vi "Get Default Value.vi"(8 "error in":errorcluster, 9 "project refnum":refnum<vi>, 10 "measurement_signature":T2, 11 "gRPCid in":T1) -> (0 "error out":errorcluster, 3 "default value":variant)   [LabVIEW 2021, in "MeasurementClient Editor.lvlib"]
uses:
  MeasurementClient Editor.lvlib
  <vilib>/gRPC/Generated APIs/ni/measurementlink/measurement/v2/Measurement Service Client V2/RPC Messages/ni_measurementlink_measurement_v2_MeasurementSignature.ctl
  <vilib>/gRPC/Generated APIs/ni/measurementlink/measurement/v2/Measurement Service Client V2/RPC Messages/ni_measurementlink_measurement_v2_ConfigurationParameter.ctl
  <vilib>/gRPC/Generated APIs/ni/measurementlink/measurement/v2/Measurement Service Client V2/RPC Messages/google_protobuf_Field_Kind.ctl
  <vilib>/gRPC/Generated APIs/ni/measurementlink/measurement/v2/Measurement Service Client V2/RPC Messages/ni_measurementlink_measurement_v2_ConfigurationParameter_AnnotationsEntry.ctl
  <vilib>/gRPC/Generated APIs/ni/measurementlink/measurement/v2/Measurement Service Client V2/RPC Messages/google_protobuf_Any.ctl
  <vilib>/gRPC/Generated APIs/ni/measurementlink/measurement/v2/Measurement Service Client V2/RPC Messages/ni_measurementlink_measurement_v2_Output.ctl
  <vilib>/gRPC/Generated APIs/ni/measurementlink/measurement/v2/Measurement Service Client V2/RPC Messages/ni_measurementlink_measurement_v2_Output_AnnotationsEntry.ctl
  <vilib>/gRPC/LabVIEW gRPC Library/Shared/grpcId.ctl
  <vilib>/Utility/traverseref.llb/TRef TravTarget.ctl
  <vilib>/gRPC/LabVIEW gRPC Library/grpc-lvsupport-release.lvlib
  <vilib>/Utility/traverseref.llb/VI Scripting - Traverse.lvlib
  <vilib>/gRPC/Generated APIs/ni/measurementlink/measurement/v2/Measurement Service Client V2/Measurement Service Client V2.lvlib
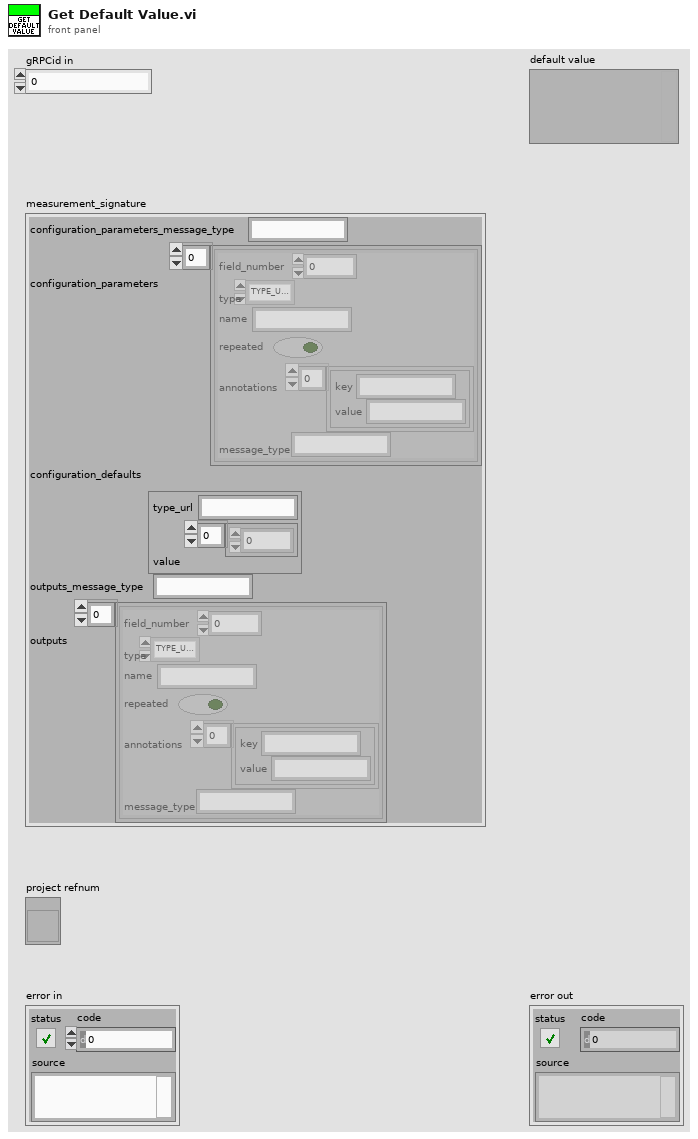
[diagram p1: front panel]
types:
  T1 = typedef "grpc-lvsupport-release.lvlib/grpcId.ctl" = u64
  T2 = typedef "Measurement Service Client V2.lvlib/ni_measurementlink_measurement_v2_MeasurementSignature.ctl" = cluster{"configuration_parameters_message_type":string, "configuration_parameters":T3[], "configuration_defaults":T6, "outputs_message_type":string, "outputs":T7[]}
  T3 = typedef "Measurement Service Client V2.lvlib/ni_measurementlink_measurement_v2_ConfigurationParameter.ctl" = cluster{"field_number":i32, "type":T4, "name":string, "repeated":bool, "annotations":T5[], "message_type":string}
  T4 = typedef "Measurement Service Client V2.lvlib/google_protobuf_Field_Kind.ctl" = enum32{"TYPE_UNKNOWN", "TYPE_DOUBLE", "TYPE_FLOAT", "TYPE_INT64", "TYPE_UINT64", "TYPE_INT32", "TYPE_FIXED64", "TYPE_FIXED32", "TYPE_BOOL", "TYPE_STRING", "TYPE_GROUP", "TYPE_MESSAGE", "TYPE_BYTES", "TYPE_UINT32", "TYPE_ENUM", "TYPE_SFIXED32", "TYPE_SFIXED64", "TYPE_SINT32", "TYPE_SINT64"}
  T5 = typedef "Measurement Service Client V2.lvlib/ni_measurementlink_measurement_v2_ConfigurationParameter_AnnotationsEntry.ctl" = cluster{"key":string, "value":string}
  T6 = typedef "Measurement Service Client V2.lvlib/google_protobuf_Any.ctl" = cluster{"type_url":string, "value":u8[]}
  T7 = typedef "Measurement Service Client V2.lvlib/ni_measurementlink_measurement_v2_Output.ctl" = cluster{"field_number":i32, "type":T4, "name":string, "repeated":bool, "annotations":T8[], "message_type":string}
  T8 = typedef "Measurement Service Client V2.lvlib/ni_measurementlink_measurement_v2_Output_AnnotationsEntry.ctl" = cluster{"key":string, "value":string}
  T9 = typedef "TRef TravTarget.ctl" = enum16{"FP", "BD", "Other"}
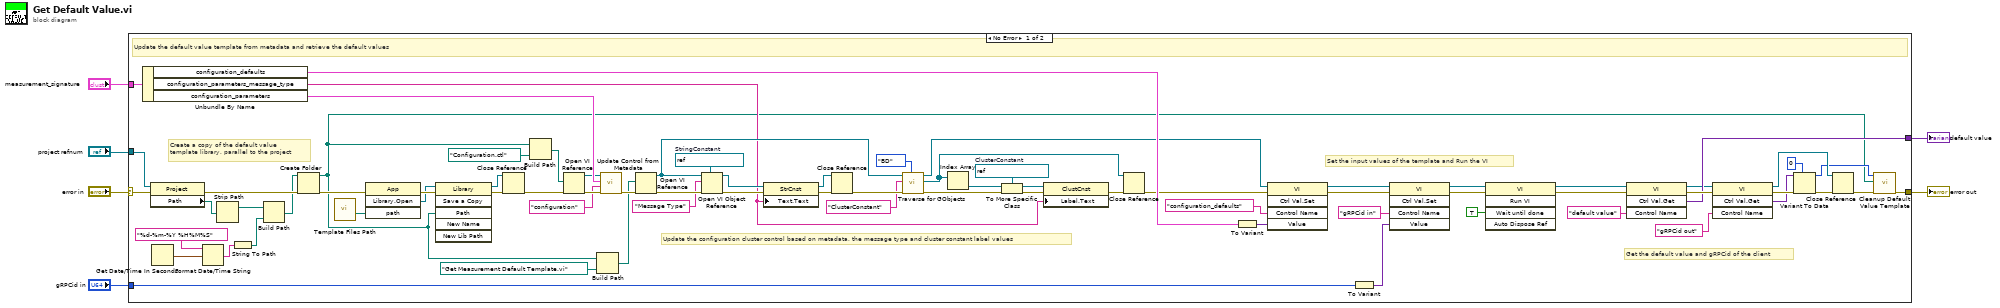
[diagram p0: block diagram]
diagram:
  n1 = case shown="No Error" "error in" {
    selector: "error in" -> [w81 w82]
    tunnel: [w10 w82] -> w5
    tunnel: "measurement_signature" -> [w11 _]
    tunnel: "gRPCid in" -> [w63 _]
    tunnel: [w54 _] -> w2
    tunnel: "project refnum" -> [w34 _]
    frame No Error {
      w39 = refnum<vi> refnum  # ClusterConstant
      w75 = refnum<vi> refnum  # StringConstant
      # "Get the default value and gRPCid of the client"
      # "Set the input values of the template and Run the VI"
      # "Update the configuration cluster control based on metadata, the message type and cluster constant label values"
      # "Create a copy of the default value\ntemplate library, parallel to the project"
      # "Update the default value template from metadata and retrieve the default values"
      n2 = Unbundle By Name(w11) -> ("configuration_defaults"=w67:T6, "configuration_parameters_message_type"=w36:string, "configuration_parameters"=w80:T3[])
      n3 = property class="Project"(reference=w34, error in=w81) -> (error out=w30:errorcluster, "Path"=w33:path)  [unwired: 1 out]
      n4 = Get Date/Time In Seconds() -> (seconds since 1Jan1904=w32:timestamp)
      n5 = Format Date/Time String(time format string (%c)="%d-%m-%Y %H%M%S", seconds (now)=w32) -> (date/time string=w21:string)  [unwired: 1 in]
      n6 = Strip Path(path=w33) -> (stripped path=w31:path)  [unwired: 1 out]
      n7 = String To Path(string=w21) -> (path=w22:path)
      n8 = Build Path(base path=w31, name or relative path=w22) -> (appended path=w28:path)
      n9 = Create Folder(path (use dialog)=w28, error in=w30) -> (created path=w8:path, error out=w29:errorcluster)  [unwired: 1 in, 1 out]
      n10 = call "Template Files Path.vi"() -> ("default template path"=w12:path)  [unwired: 9 in, 2 out]
      n11 = invoke class="App" method="Library.Open"(error in=w29, "path"=w12) -> (error out=w18:errorcluster, "Open Library"=w16:refnum<vi>)  [unwired: 2 in, 2 out]
      n12 = invoke class="Library" method="Save a Copy"(reference=w16, error in=w18, "Path"=w8) -> (reference out=w13:refnum<vi>, error out=w17:errorcluster)  [unwired: 3 in, 4 out]
      n13 = Close Reference(reference=w13, error in (no error)=w17) -> (error out=w14:errorcluster)
      n14 = Build Path(base path=w8, name or relative path=path "Configuration.ctl") -> (appended path=w26:path)
      n15 = Open VI Reference(vi path=w26, error in (no error)=w14) -> (vi reference=w25:refnum<vi>, error out=w27:errorcluster)  [unwired: 4 in]
      n16 = Build Path(base path=w8, name or relative path=path "Get Measurement Default Template.vi") -> (appended path=w23:path)
      n17 = call "Update Control from Metadata.vi"("error in"=w27, "control name"="configuration", "parameter data"=w80, "vi refnum"=w25) -> ("error out"=w79:errorcluster)  [unwired: 7 in]
      n18 = Open VI Reference(vi path=w23, error in (no error)=w79) -> (vi reference=w43:refnum<vi>, error out=w78:errorcluster)  [unwired: 4 in]
      n19 = Open VI Object Reference(7:w75, 8:w78, 10:"Message Type" ("name/order"), 11:w43) -> (0:w76:errorcluster, 3:w73:refnum<vi>)
      n20 = property class="StrCnst"(reference=w73, error in=w76, "Text.Text"=w36) -> (reference out=w72:refnum<vi>, error out=w74:errorcluster)
      n21 = Close Reference(reference=w72, error in (no error)=w74) -> (error out=w71:errorcluster)
      n22 = call <vilib>:"Traverse for GObjects.vi"("Traverse Target"=TRef_TravTarget."BD", "error in (no error)"=w71, "Class Name"="ClusterConstant", "VI Refnum"=w43) -> ("error out"=w40:errorcluster, "References"=w7:refnum<vi>[], "dup VI Refnum"=w46:refnum<vi>)  [unwired: 4 in, 1 out]
      n23 = Index Array(array=w7) -> (element=w38:refnum<vi>)  [unwired: 1 in]
      n24 = To More Specific Class(target class=w39, reference=w38, error in=w40) -> (specific class reference=w37:refnum<vi>, error out=w41:errorcluster)
      n25 = property class="ClustCnst"(reference=w37, error in=w41, "Label.Text"=w36) -> (error out=w42:errorcluster)  [unwired: 1 out]
      n26 = Close Reference(reference=w7, error in (no error)=w42) -> (error out=w35:errorcluster)
      n27 = To Variant(anything=w67) -> (Variant=w66:variant)
      n28 = invoke class="VI" method="Ctrl Val.Set"(reference=w46, error in=w35, "Control Name"="configuration_defaults", "Value"=w66) -> (reference out=w64:refnum<vi>, error out=w69:errorcluster)  [unwired: 1 in, 3 out]
      n29 = To Variant(anything=w63) -> (Variant=w62:variant)
      n30 = invoke class="VI" method="Ctrl Val.Set"(reference=w64, error in=w69, "Control Name"="gRPCid in", "Value"=w62) -> (reference out=w59:refnum<vi>, error out=w65:errorcluster)  [unwired: 1 in, 3 out]
      n31 = invoke class="VI" method="Run VI"(reference=w59, error in=w65, "Wait until done"=TRUE ("Wait Until Done")) -> (reference out=w56:refnum<vi>, error out=w60:errorcluster)  [unwired: 2 in, 3 out]
      n32 = invoke class="VI" method="Ctrl Val.Get"(reference=w56, error in=w60, "Control Name"="default value") -> (reference out=w52:refnum<vi>, error out=w57:errorcluster, "Get Control Value Variant"=w54:variant)  [unwired: 1 in, 1 out]
      n33 = invoke class="VI" method="Ctrl Val.Get"(reference=w52, error in=w57, "Control Name"="gRPCid out") -> (reference out=w48:refnum<vi>, error out=w53:errorcluster, "Get Control Value Variant"=w49:variant)  [unwired: 1 in, 1 out]
      n34 = Variant To Data(error in=w53, type=T1 0 ("gRPCid in"), Variant=w49) -> (data=w9:T1, error out=w50:errorcluster)
      n35 = Close Reference(reference=w48, error in (no error)=w50) -> (error out=w70:errorcluster)
      n36 = call "Cleanup Default Value Template.vi"("error in"=w70, "temporary template path"=w8, "gRPCid in"=w9) -> ("error out"=w10:errorcluster)  [unwired: 8 in]
    }
    frame Error {
      # "Pass"
    }
  }
  "error out" <- w5
  "default value" <- w2
